vi "Intan_StreamData_64ch_parallelLoop_ambulatory.vi"(0 "VISA resource name":refnum<visa-resource-name>, 1 "refnum in":refnum<file>, 3 "stop streaming":bool, 4 "Save Binary Data":bool, 5 "error in":errorcluster, 7 "byte order":T5(ring)=enum."little-endian", 8 "hdr fpath":path, 11 "DT_scale (sec)":dbl=0.01, 12 "aux file ref num":refnum<file>, 14 "save aux file":bool) -> (6 "N data scans to read (VISA)":i32=20, 10 "Nbytes VISA read":u32, 13 "VISA read iter":i32, 19 "error out":errorcluster)   [LabVIEW 2017]
doc: "Stream data to disk and user friendly display. Data is scaled and filtered prior to display.\n\nThis VI uses parallel while loop architecture: 1 loop reads from serial stream and saves raw bytes to disk; the other loop processes the data in chunk, scaling and filtering, then displays."
uses:
  zip_swcircularbuffer1_0_19b/Circular Buffer/Controls/Circular Buffer Status.ctl
  zip_swcircularbuffer1_0_19b/Circular Buffer/Controls/Circular Buffer Operations.ctl
  <vilib>/Utility/error.llb/DialogType.ctl
  zip_swcircularbuffer1_0_19b/Circular Buffer/Instance VIs/Circular Buffer(1D U16).vi
  zip_swcircularbuffer1_0_19b/Circular Buffer/Circular Buffer.lvlib
panel:
  out "ADXL Stream":dbl[][](graph)
  out "A+B chans":i32[](array[numeric])
  out "Bchans":i32[](array[numeric])
  out "Achans":i32[](array[numeric])
  in  "Tab Control":T1(tab)
  in  "stop logging":bool
  in  "DisplayScale (uV/div)":u16(ring)=1 items=["6400", "3200", "1600", "800", "400", "200", "100", "50", "25"]
  in  "offset factor":dbl=1.0
  in  "Filter settings":T2={"LP Filter On/Off"=TRUE, "LP Cutoff (Hz)"=40.0, "HP Filter On/Off"=TRUE, "HP Cutoff (Hz)"=0.5, "Bandstop On/Off"=TRUE, "fl Cutoff (Hz)"=48.0, "fh Cutoff (Hz) "=52.0}
  out "Save status":bool
  out "non integer read":bool
  out "display iter":i32
  out "% buffer full":dbl(slide) scale=0.0..100.0
  in  "Ring Buffer Size":T3={"Samples per Channel"=640000, "Channels"=0}
  out "buffer underflow":bool
  out "Buffer Status  (read)":T4
  out "buffer overflow":bool
  out "Buffer Status (write)":T4
  in  "Center Traces":bool
  in  "Display Chans":i32[](listbox)=[1, 4, 13, 14, 15, 16, 17, 22]
  out "FS (Hz)":dbl
  in  "ChartDisplayLength (s)":dbl=5.0
  in  "Display Update interval (ms)":dbl=100.0
  in  "Buffer Read Interval (ms)":dbl=100.0
  in  "View Channels":u16(ring) items=["A and B (0-63)", "A chans (0-31)", "B chans (32-63)", "Free Select"]
  in  "bytes per scan":i32=148
  in  "Nchans":i32=64
  in  "start stream (Teensy char)":string="s"
  in  "stop serial stream (Teensy char)":string="t"
  out "Text response":string
  out "timestamp_array":i32[](array[numeric])
  out "aux_cmd_array":i32[][](array[numeric])
  out "binary data (from VISA read)":u16[](array[numeric])
  out "SyncBytes Out":i32[](array[numeric])
  in  "stop logging Teensy char":string="l"
  out "setscaleresult":dbl
  out "UpdateCode":i16
  out "xmax_init":dbl
  out "offset_init":dbl
  out "increment_init":dbl
  out "xmin_init":dbl
  out "NchansChanged":bool
  out "DispLengthChanged":bool
  out "XscaleRollover":bool
  out "error code out":i32 format="%0.0f"
  out "StopLoopsMaster":bool
  out "N_u16s  write to buf":i32
  out "Nelements to read from buf":dbl
  out "N data scans to display":u16=20
  out "YtxtLabelsAll":string[](array[string])
  out "Picture":picture
  out "Intan Streaming Data":dbl[][](graph)
  # "Intan-Teensy Bioelectric Module: Data Stream and Visualization\n64 chan + ADXL"
  # "Data Streaming Frequency"
  # "Display Settings"
  # "Ring Buffer Status"
  # "1-D data stream \nreformatted  to 2-D"
  # "xscale controls"
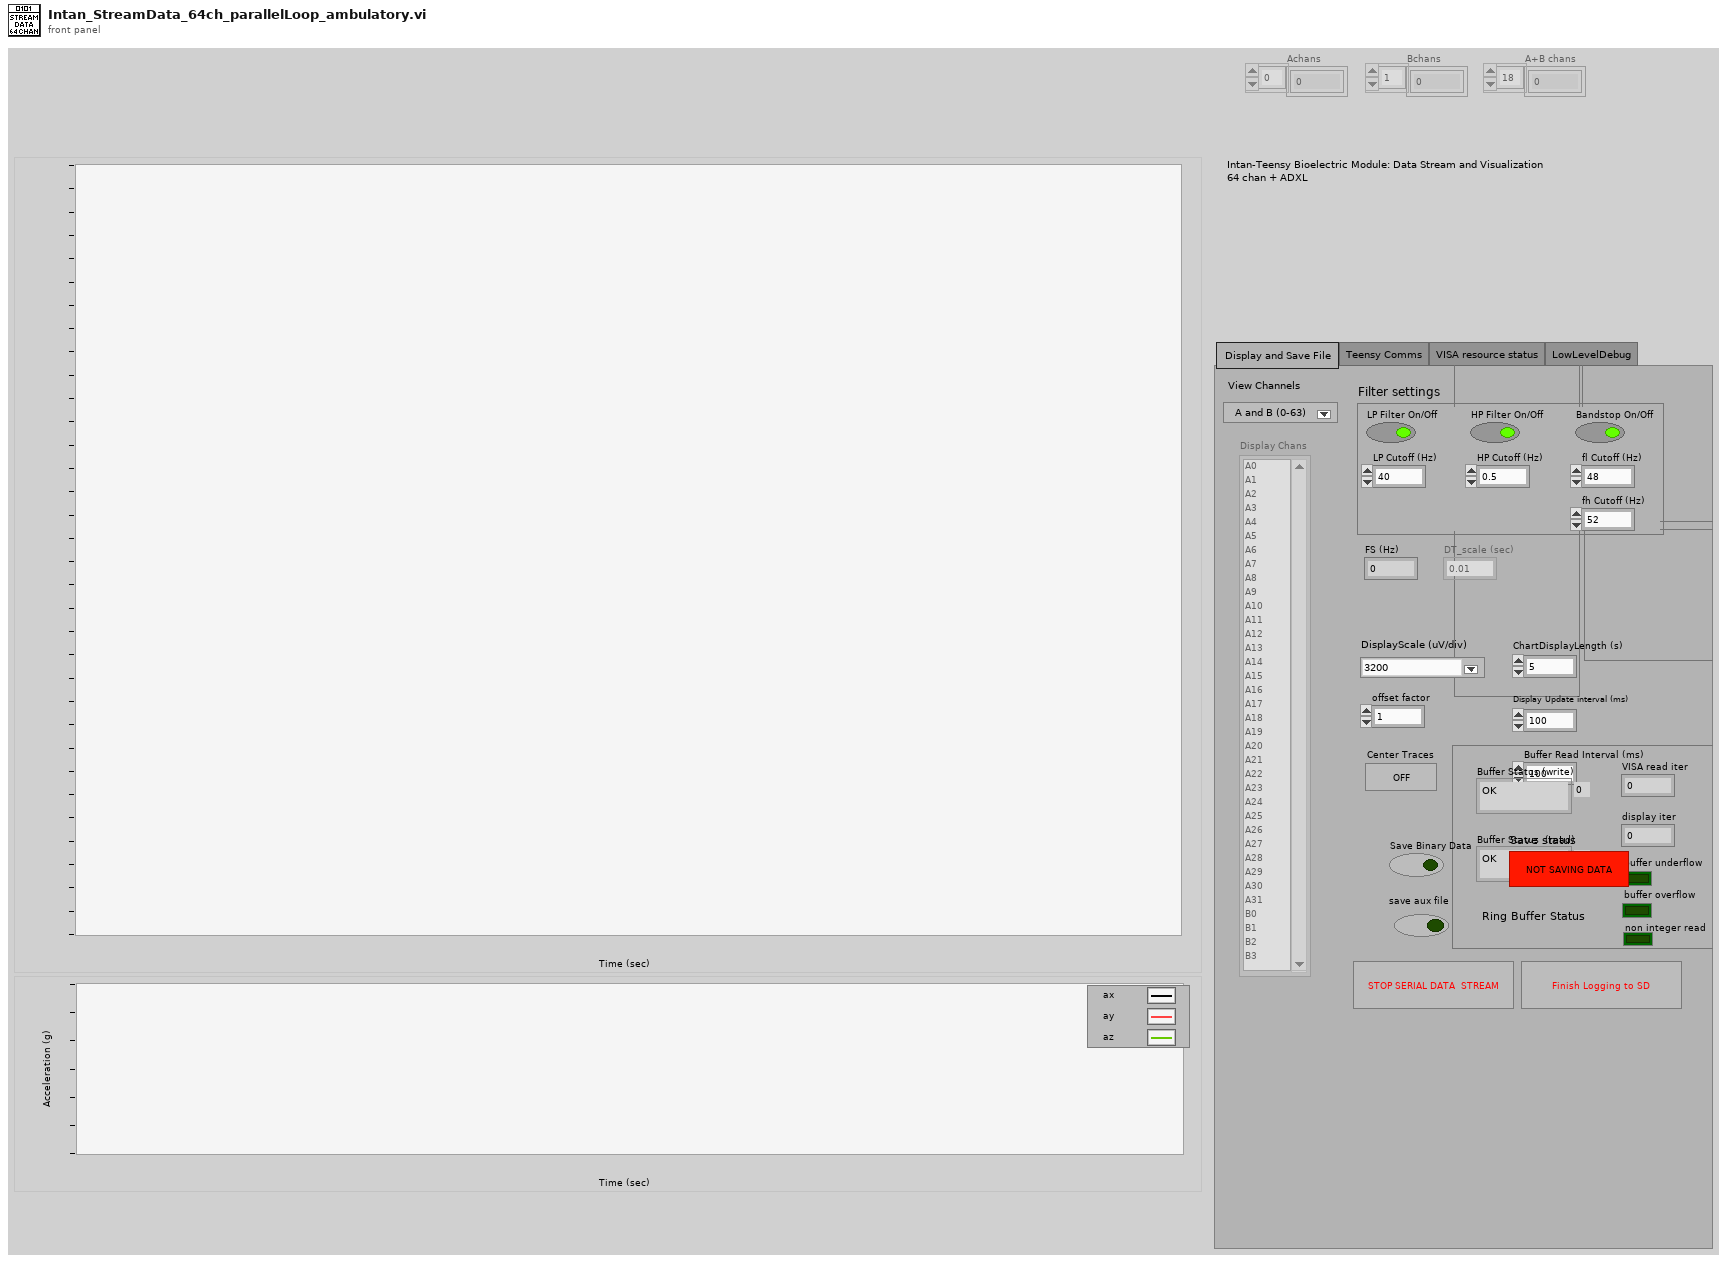
[diagram p1: front panel]
types:
  T1 = enum32{"Display and Save File ", "Teensy Comms", "VISA resource status", "LowLevelDebug"}
  T2 = cluster{"LP Filter On/Off":bool, "LP Cutoff (Hz)":dbl, "HP Filter On/Off":bool, "HP Cutoff (Hz)":dbl, "Bandstop On/Off":bool, "fl Cutoff (Hz)":dbl, "fh Cutoff (Hz) ":dbl}
  T3 = cluster{"Samples per Channel":u32, "Channels":u32}
  T4 = typedef "Circular Buffer.lvlib/Circular Buffer Status.ctl" = enum16{"OK", "Overflow", "Underflow"}
  T5 = enum16{"big-endian, network order", "native, host order", "little-endian"}
  T6 = typedef "Circular Buffer.lvlib/Circular Buffer Operations.ctl" = enum16{"Initialize", "Get Backlog", "Write", "Read (continuous)", "Read (most recent)"}
  T7 = enum8{"Enabled", "Disabled", "Disabled and Grayed Out"}
  T8 = typedef "LVRectTypeDef.ctl" = cluster{"Left":i16, "Top":i16, "Right":i16, "Bottom":i16}
  T9 = cluster{"XScale.Minimum":dbl, "XScale.Maximum":dbl, "XScale.Increment":dbl, "Nchannels":i32}
  T10 = cluster{"Maximum":dbl, dbl, dbl, dbl, dbl, dbl, "YscleMark":dbl, "Increment":dbl}
  T11 = typedef "DialogType.ctl" = u16
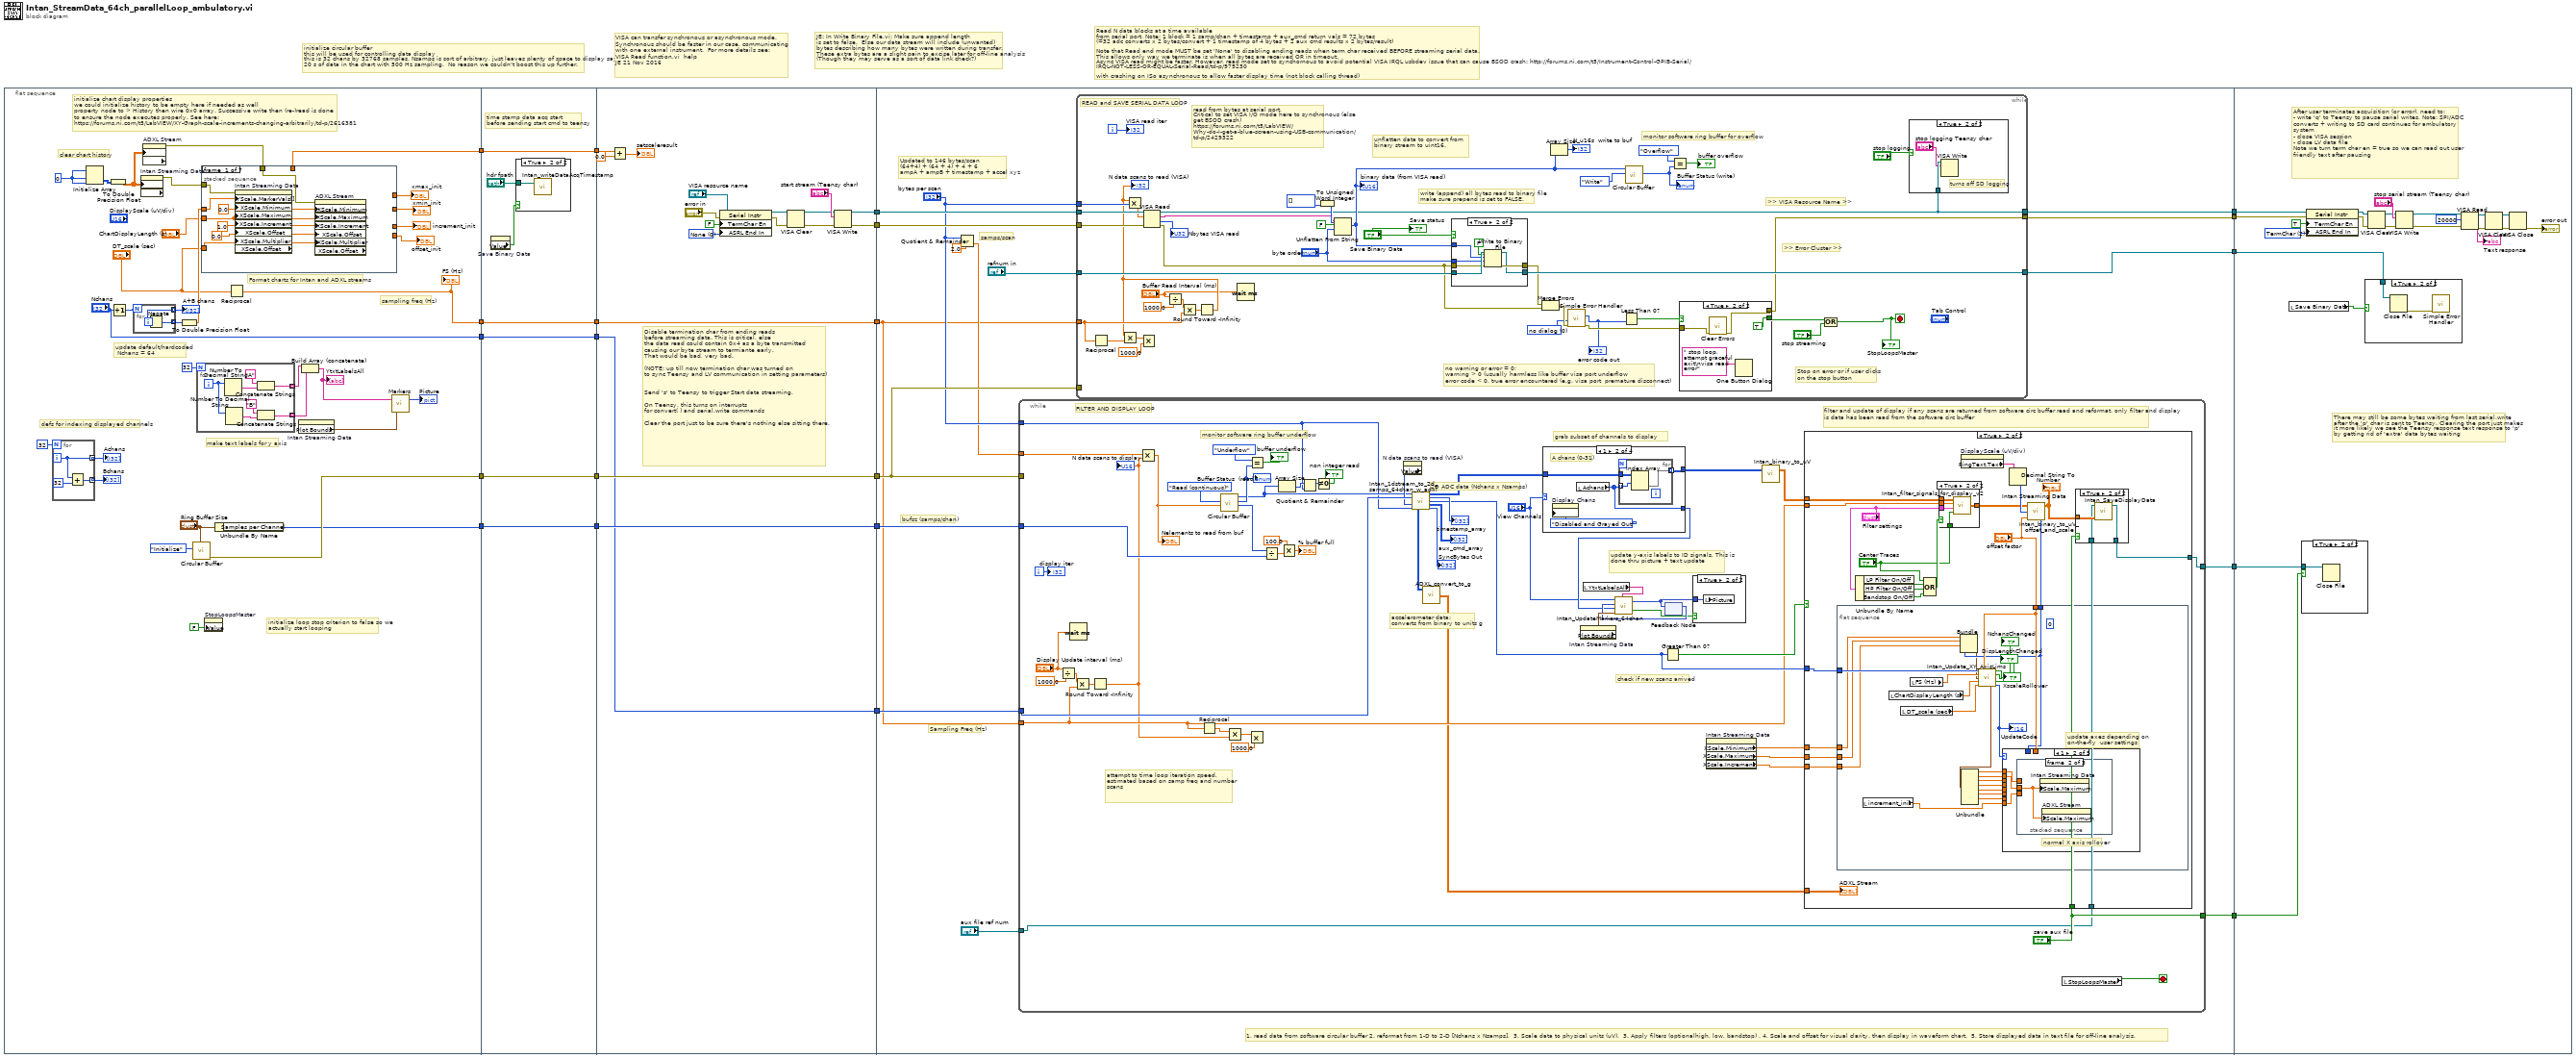
[diagram p0: block diagram]
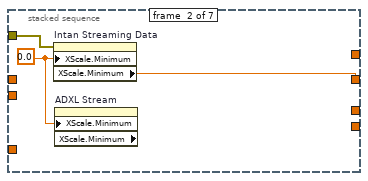
[diagram p2: hidden frame]
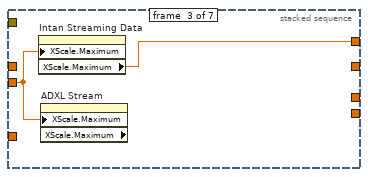
[diagram p3: hidden frame]
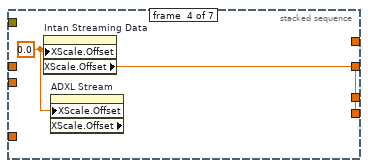
[diagram p4: hidden frame]
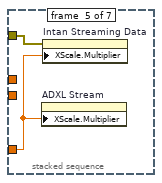
[diagram p5: hidden frame]
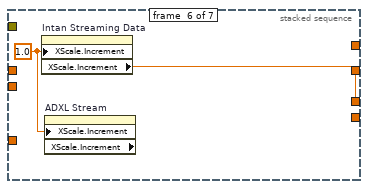
[diagram p6: hidden frame]
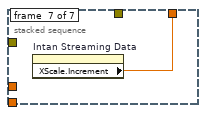
[diagram p7: hidden frame]
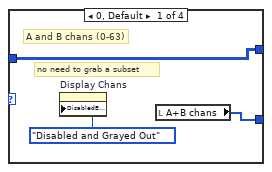
[diagram p10: hidden frame]
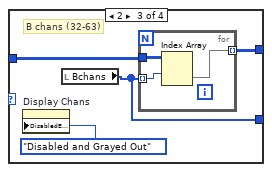
[diagram p11: hidden frame]
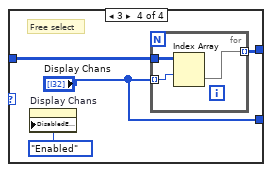
[diagram p12: hidden frame]
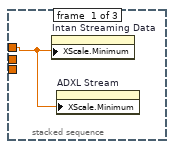
[diagram p15: hidden frame]
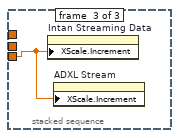
[diagram p16: hidden frame]
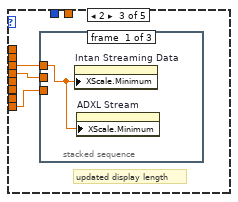
[diagram p17: hidden frame]
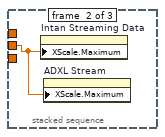
[diagram p18: hidden frame]
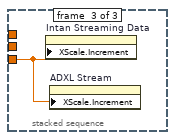
[diagram p19: hidden frame]
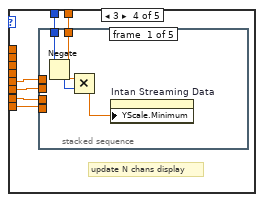
[diagram p20: hidden frame]
diagram:
  # "Read N data blocks at a time available\nfrom serial port. Note: 1 block = 1 samp/chan + timestamp + aux_cmd return vals = 72 bytes \n(=32 adc converts x 2 bytes/convert + 1 timestamp of 4 bytes + 2 aux cmd results x 2 bytes/result) \n\nNote that Read end mode MUST be set 'None' to disabling ending reads when term char received BEFORE streaming serial data.  \nThis allows only way we terminate is when all bytes are received OR in timeout.  \nAsync VISA read might be faster. However, read mode set to synchornous to avoid potential VISA IRQL usbdev issue that can cause BSOD crash: http://forums.ni.com/t5/Instrument-Control-GPIB-Serial/IRQL-NOT-LESS-OR-EQUAL-Serial-Read/td-p/975230\n\nwith crashing on ISo asynchronous to allow faster display time (not block calling thread)"
  # "initialize circular buffer\nthis will be used for controlling data display\nthis is 32 chans by 32768 samples. Nsamps is sort of arbitrary, just leaves plenty of space to display say\n20 s of data in the chart with 500 Hz sampling.  No reason we couldn't boost this up further."
  # "JE: In Write Binary File.vi: Make sure append length \nis set to false.  Else our data stream will include (unwanted)\nbytes describing how many bytes were written during transfer.\nThese extra bytes are a slight pain to excise later for off-line analysis\n(Though they may serve as a sort of data link check?)"
  # "VISA can transfer synchronous or asynchronous mode.\nSynchronous should be faster in our case, communicating\nwith one external instrument.  For more details see: \nVISA Read function.vi  help \nJE 21 Nov 2016"
  n1 = flat-sequence {
    tunnel: [w50] -> w10
    tunnel: [w48] -> w8
    tunnel: ["Nchans"] -> w6
    tunnel: [w43] -> w4
    tunnel: [w32] -> w2
    tunnel: w10 -> [w92]
    tunnel: [w92] -> w9
    tunnel: w8 -> [w91]
    tunnel: [w91] -> w7
    tunnel: w6 -> [w90]
    tunnel: [w90] -> w5
    tunnel: w4 -> [w89]
    tunnel: [w89] -> w3
    tunnel: w2 -> [w88]
    tunnel: [w88] -> w1
    tunnel: [w101] -> w19
    tunnel: [w102] -> w18
    tunnel: [w100] -> w17
    tunnel: w9 -> [w100]
    tunnel: [w99] -> w16
    tunnel: w7 -> [w99]
    tunnel: w5 -> [w98]
    tunnel: [w98] -> w15
    tunnel: [w97] -> w14
    tunnel: w3 -> [w97]
    tunnel: w1 -> [w96]
    tunnel: [w123] -> w21
    tunnel: [w126] -> w20
    tunnel: w19 -> [w124]
    tunnel: w18 -> [w125]
    tunnel: w17 -> [w122]
    tunnel: w16 -> [w120]
    tunnel: w15 -> [w119]
    tunnel: w14 -> [w116]
    tunnel: [w115] -> w13
    tunnel: [w113] -> w12
    tunnel: [w112] -> w11
    tunnel: w21 -> [w370]
    tunnel: w20 -> [w383]
    tunnel: w13 -> [w365]
    tunnel: w12 -> [w364]
    tunnel: w11 -> [w363]
    frame #0 {
      w42 = 0 ("Dimension Size")
      # "Format charts for Intan and ADXL streams"
      # "defs for indexing displayed channels"
      # "update default/hardcoded\n Nchans = 64"
      # "clear chart history"
      # "initialize loop stop criterion to false so we\nactually start looping"
      # "make text labels for y axis"
      # "sampling freq (Hz)"
      # "initialize chart display properties\nwe could initialize history to be empty here if needed as well\nproperty node to > History then wire 0x0 array. Successive write then (re-)read is done\nto ensure the node executes properly. See here:\nhttps://forums.ni.com/t5/LabVIEW/XY-Graph-scale-increments-changing-arbitrarily/td-p/2616381"
      n2 = for {
        N: 32 -> [_]
        tunnel: [w56] -> w30 mode=indexing
        tunnel: [w54] -> w29 mode=indexing
        i -> [w56]
        n3 = Add(x=w56, y=32) -> (x+y=w54:i32)
      }
      "Achans" <- w30
      "Bchans" <- w29
      n4 = Initialize Array(w42, w42, w42) -> (w41:i32[][])
      n5 = To Double Precision Float(number=w41) -> (double precision float=w23:dbl[][])
      n6 = Increment(x="Nchans") -> (x+1=w52:i32)
      n7 = for {
        N: w52 -> [_]
        tunnel: [w85] -> w53 mode=indexing
        tunnel: [w84] -> w28 mode=indexing
        i -> [w84]
        n8 = Negate(x=w84) -> (-x=w85:i32)
      }
      "A+B chans" <- w28
      n9 = property on="Intan Streaming Data" class="WFChart (strict)" props=["History Data", "History Data"]("History Data"=w23) -> (error out=w39:errorcluster)  [unwired: 2 in, 2 out]
      n10 = property on="ADXL Stream" class="WFChart (strict)" props=["History Data", "History Data"]("History Data"=w23) -> (error out=w22:errorcluster)  [unwired: 2 in, 2 out]
      n11 = To Double Precision Float(number=w53) -> (double precision float=w40:dbl[])
      n12 = call-poly "Circular Buffer.vi"("Buffer Size"="Ring Buffer Size", "Operation"=Circular_Buffer_Operations."Initialize") -> ("error out"=w50:errorcluster)  [unwired: 6 in, 3 out]
      n13 = for {
        N: 32 -> [_]
        tunnel: [w81] -> w26 mode=indexing
        tunnel: [w77] -> w25 mode=indexing
        i -> [w78]
        n14 = Number To Decimal String(number=w78) -> (decimal integer string=w83:string)  [unwired: 1 in]
        n15 = Number To Decimal String(number=w78) -> (decimal integer string=w80:string)  [unwired: 1 in]
        n16 = Concatenate Strings("A" ("string"), w83) -> (w81:string)
        n17 = Concatenate Strings("B" ("string"), w80) -> (w77:string)
      }
      n18 = stacked-sequence {
        tunnel: w40 -> [w64 _ _ _ _ _ _]
        tunnel: w39 -> [w63 w66 _ _ w73 _ _]
        tunnel: "ChartDisplayLength (s)" -> [w61 _ w68 _ _ _ _]
        tunnel: "DT_scale (sec)" -> [w58 _ _ _ w72 _ _]
        tunnel: [_ _ w69 _ _ _ _] -> w33
        tunnel: [_ w67 _ _ _ _ _] -> w36
        tunnel: [_ _ _ _ _ w75 _] -> w35
        tunnel: [_ _ _ w71 _ _ _] -> w34
        tunnel: [_ _ _ _ _ _ w76] -> w32
        tunnel: w22 -> [w57 _ _ _ _ _ _]
        frame #0 {
          w60 = 1.0 ("X Scale.Range:Minimum")
          w59 = 0.0 ("X Scale.Range:Minimum")
          w62 = 0.0 ("X Scale.Range:Minimum")
          n19 = property on="Intan Streaming Data" class="WFChart (strict)" props=["YScale", "MarkerVals[]", "XScale", "Minimum", "XScale", "Maximum", "XScale", "Increment", "XScale", "Offset", "XScale", "Multiplier", "XScale", "Offset"](error in=w63, "YScale.MarkerVals[]"=w64, "XScale.Minimum"=w62, "XScale.Maximum"=w61, "XScale.Increment"=w60, "XScale.Offset"=w59, "XScale.Multiplier"=w58) -> ()  [unwired: 1 in, 3 out]
          n20 = property on="ADXL Stream" class="WFChart (strict)" props=["XScale", "Minimum", "XScale", "Maximum", "XScale", "Increment", "XScale", "Offset", "XScale", "Multiplier", "XScale", "Offset"](error in=w57, "XScale.Minimum"=w62, "XScale.Maximum"=w61, "XScale.Increment"=w60, "XScale.Offset"=w59, "XScale.Multiplier"=w58) -> ()  [unwired: 1 in, 3 out]
        }
        frame #1 {
          w65 = 0.0 ("X Scale.Range:Minimum")
          n21 = property on="Intan Streaming Data" class="WFChart (strict)"(error in=w66, "XScale.Minimum"=w65) -> ("XScale.Minimum"=w67:dbl)  [unwired: 1 in, 2 out]
          n22 = property on="ADXL Stream" class="WFChart (strict)" props=["XScale", "Minimum", "XScale", "Minimum"]("XScale.Minimum"=w65) -> ()  [unwired: 2 in, 3 out]
        }
        frame #2 {
          n23 = property on="Intan Streaming Data" class="WFChart (strict)"("XScale.Maximum"=w68) -> ("XScale.Maximum"=w69:dbl)  [unwired: 2 in, 2 out]
          n24 = property on="ADXL Stream" class="WFChart (strict)" props=["XScale", "Maximum", "XScale", "Maximum"]("XScale.Maximum"=w68) -> ()  [unwired: 2 in, 3 out]
        }
        frame #3 {
          w70 = 0.0 ("X Scale.Offset and Multiplier:Offset")
          n25 = property on="Intan Streaming Data" class="WFChart (strict)"("XScale.Offset"=w70) -> ("XScale.Offset"=w71:dbl)  [unwired: 2 in, 2 out]
          n26 = property on="ADXL Stream" class="WFChart (strict)" props=["XScale", "Offset", "XScale", "Offset"]("XScale.Offset"=w70) -> ()  [unwired: 2 in, 3 out]
        }
        frame #4 {
          n27 = property on="ADXL Stream" class="WFChart (strict)"("XScale.Multiplier"=w72) -> ()  [unwired: 2 in, 2 out]
          n28 = property on="Intan Streaming Data" class="WFChart (strict)"(error in=w73, "XScale.Multiplier"=w72) -> ()  [unwired: 1 in, 2 out]
        }
        frame #5 {
          w74 = 1.0 ("X Scale.Range:Increment")
          n29 = property on="Intan Streaming Data" class="WFChart (strict)"("XScale.Increment"=w74) -> ("XScale.Increment"=w75:dbl)  [unwired: 2 in, 2 out]
          n30 = property on="ADXL Stream" class="WFChart (strict)" props=["XScale", "Increment", "XScale", "Increment"]("XScale.Increment"=w74) -> ()  [unwired: 2 in, 3 out]
        }
        frame #6 {
          n31 = property on="Intan Streaming Data" class="WFChart (strict)"() -> ("XScale.Increment"=w76:dbl)  [unwired: 2 in, 2 out]
        }
      }
      "xmin_init" <- w36
      "increment_init" <- w35
      "offset_init" <- w34
      "xmax_init" <- w33
      n32 = property on="StopLoopsMaster" class="Bool (strict)"("Value"=FALSE ("StopLoopsMaster")) -> ()  [unwired: 2 in, 2 out]
      n33 = Unbundle By Name("Ring Buffer Size") -> ("Samples per Channel"=w48:u32)
      n34 = Reciprocal(x="DT_scale (sec)") -> (1/x=w43:dbl)
      "FS (Hz)" <- w43
      n35 = property on="Intan Streaming Data" class="WFChart (strict)"() -> ("Plot Bounds"=w44:T8)  [unwired: 2 in, 2 out]
      n36 = Build Array (concatenate)(w26, w25) -> (w24:string[])
      "YtxtLabelsAll" <- w24
      n37 = call "Markers.vi"("plot bounds"=w44, "Array"=w24) -> ("Picture"=→"Picture":picture)  [unwired: 1 out]
    }
    frame #1 {
      # "time stamp data acq start\nbefore sending start cmd to teensy"
      n38 = property on="Save Binary Data" class="Bool (strict)"() -> ("Value"=w87:bool)  [unwired: 2 in, 2 out]
      n39 = case shown="True" w87 {
        tunnel: "hdr fpath" -> [_ w93]
        frame False {
        }
        frame True {
          n40 = call "Intan_writeDataAcqTimestamp.vi"("hdr fpath"=w93) -> ()  [unwired: 2 in, 1 out]
        }
      }
    }
    frame #2 {
      w107 = u16 0 items=["None", "Last Bit", "TermChar"] ("Serial Settings:End Mode for Reads")
      # "Disable termination char from ending reads\nbefore streaming data. This is critical, else\nthe data read could contain 0x4 as a byte transmitted\ncausing our byte stream to termiante early.\nThat would be bad, very bad.\n\n(NOTE: up till now termination char was turned on\nto sync Teensy and LV communication in setting parameters)\n\n\nSend 's' to Teensy to trigger Start data streaming.  \n\nOn Teensy, this turns on interrupts\nfor convert( ) and serial.write commands\n\nClear the port just to be sure there's nothing else sitting there."
      n41 = Add(x=w96, y=0.0) -> (x+y=→"setscaleresult":dbl)
      n42 = property class="Serial Instr"(reference="VISA resource name", error in="error in", "TermChar En"=FALSE ("Message Based Settings:Termination Character Enable"), "ASRL End In"=w107) -> (reference out=w106:refnum<visa-resource-name>, error out=w105:errorcluster)
      n43 = VISA Clear(VISA resource name=w106, error in (no error)=w105) -> (VISA resource name out=w104:refnum<visa-resource-name>, error out=w103:errorcluster)
      n44 = VISA Write(VISA resource name=w104, write buffer="start stream (Teensy char)", error in (no error)=w103) -> (VISA resource name out=w102:refnum<visa-resource-name>, error out=w101:errorcluster)  [unwired: 1 out]
    }
    frame #3 {
      # "Updated to 146 bytes/scan\n(64+4) + (64 + 4) + 4 + 6\nampA + ampB + timestamp + accel xyz"
      # "1. read data from software circular buffer 2. reformat from 1-D to 2-D [Nchans x Nsamps].  3. Scale data to physical units (uV).  3. Apply filters (optionalhigh, low, bandstop) . 4. Scale and offset for visual clarity, then display in waveform chart.  5. Store displayed data in text file for off-line analysis."
      # "Sampling Freq (Hz)"
      # "bufsz (samps/chan)"
      # "samps/scan"
      n45 = Quotient & Remainder(x="bytes per scan", y=2.0) -> (floor(x/y)=w117:dbl)  [unwired: 1 out]
      n46 = while {
        tunnel: w122 -> [_]
        tunnel: w120 -> [w174]
        tunnel: w119 -> [w170]
        tunnel: "bytes per scan" -> [w160]
        tunnel: w116 -> [w141]
        tunnel: w117 -> [w166]
        tunnel: [w147] -> w115
        tunnel: "aux file ref num" -> [w146]
        tunnel: ["save aux file"] -> w112
        i -> [w167]
        stop <- w144 stop-if-true
        # "accelerometer data: \nconverts from binary to units g"
        # "2D ADC data (Nchans x Nsamps)"
        # "check if new scans arrived"
        # "grab subset of channels to display"
        # "update y-axis labels to ID signals. This is done thru picture + text update"
        # "FILTER AND DISPLAY LOOP"
        # "attempt to time loop iteration speed,\nestimated based on samp freq and number scans"
        # "filter and update of display if any scans are returned from software circ buffer read and reformat. only filter and display is data has been read from the software circ buffer"
        # "monitor software ring buffer underflow"
        n47 = Divide(x="Display Update interval (ms)", y=1000.0) -> (x/y=w138:dbl)
        n48 = Wait (ms)(milliseconds to wait="Display Update interval (ms)") -> ()  [unwired: 1 out]
        n49 = Multiply(x=w138, y=w141) -> (x*y=w140:dbl)
        n50 = Round Toward -Infinity(1:w140) -> (0:w139:dbl)
        "N data scans to display" <- w139
        n51 = Multiply(x=w166, y=w139) -> (x*y=w165:dbl)
        "Nelements to read from buf" <- w165
        n52 = Reciprocal(x=w141) -> (1/x=w157:dbl)
        n53 = call-poly "Circular Buffer.vi"("Read Size"=w165, "Operation"=Circular_Buffer_Operations."Read (continuous)") -> ("Elements Remaining"=w175:i32, "Buffer Status"=w177:T4, "Data Out"=w162:u16[])  [unwired: 6 in, 1 out]
        "Buffer Status  (read)" <- w177
        n54 = Multiply(x=w157, y=w139) -> (x*y=w156:dbl)
        n55 = Multiply(x=w156, y=1000.0) -> ()  [unwired: 1 out]
        n56 = Equal?(x=Circular_Buffer_Status."Underflow" ("y"), y=w177) -> (x = y?=→"buffer underflow":bool)
        n57 = Divide(x=w175, y=w174) -> (x/y=w173:dbl)
        n58 = Array Size(array=w162) -> (size(s)=w161:i32)
        n59 = Multiply(x=100.0, y=w173) -> (x*y=→"% buffer full":dbl)
        n60 = Quotient & Remainder(x=w161, y=w160) -> (x-y*floor(x/y)=w159:i32)  [unwired: 1 out]
        n61 = Not Equal To 0?(x=w159) -> (x != 0?=→"non integer read":bool)
        n62 = property on="N data scans to read (VISA)" class="DigNum (strict)"() -> ("Value"=w164:i32)  [unwired: 2 in, 2 out]
        n63 = call "Intan_1dstream_to_2d_samps_64chan_w_adxl.vi"("1-D  data in"=w162, "Nchans"=w170, "N data scans to read"=w164, "bytes per scan"=w160) -> ("2d ADCdata_array out_ampA_and_B"=w154:u16[][], "timestamp_array"=→"timestamp_array":i32[], "Nscans read"=w145:i32, "aux_cmd_array A_and_B"=→"aux_cmd_array":i16[][], "ADXL analog data out"=w130:u16[][], "SyncBytes Out"=→"SyncBytes Out":i32[])  [unwired: 4 in, 2 out]
        n64 = call "ADXL_convert_to_g.vi"("ADXL analog data out: Binary format"=w130) -> ("ADXL scaled (units of g)"=w129:dbl[][])  [unwired: 3 in]
        n65 = case shown="1" "View Channels" {
          tunnel: w154 -> [w183 w187 w194 w201]
          tunnel: [w183 w186 w193 w200] -> w143
          tunnel: [w181 w184 w191 "Display Chans"] -> w132
          frame 0, Default {
            # "A and B chans (0-63)"
            # "no need to grab a subset"
            n66 = property on="Display Chans" class="LstBox (strict)"("DisabledEnum"=T7."Disabled and Grayed Out" ("Disabled")) -> ()  [unwired: 2 in, 2 out]
            n67 = local read "A+B chans"() -> (w181:i32[])
          }
          frame 1 {
            # "A chans (0-31)"
            n68 = property on="Display Chans" class="LstBox (strict)"("DisabledEnum"=T7."Disabled and Grayed Out" ("Disabled")) -> ()  [unwired: 2 in, 2 out]
            n69 = local read "Achans"() -> (w184:i32[])
            n70 = for {
              tunnel: w187 -> [w190]
              tunnel: w184 -> [w188] mode=indexing
              tunnel: [w189] -> w186 mode=indexing
              n71 = Index Array(array=w190, index (row)=w188) -> (element=w189:u16[])  [unwired: 1 in]
            }
          }
          frame 2 {
            # "B chans (32-63)"
            n72 = property on="Display Chans" class="LstBox (strict)"("DisabledEnum"=T7."Disabled and Grayed Out" ("Disabled")) -> ()  [unwired: 2 in, 2 out]
            n73 = local read "Bchans"() -> (w191:i32[])
            n74 = for {
              tunnel: w194 -> [w197]
              tunnel: w191 -> [w195] mode=indexing
              tunnel: [w196] -> w193 mode=indexing
              n75 = Index Array(array=w197, index (row)=w195) -> (element=w196:u16[])  [unwired: 1 in]
            }
          }
          frame 3 {
            # "Free select"
            n76 = property on="Display Chans" class="LstBox (strict)"("DisabledEnum"=T7."Enabled" ("Disabled")) -> ()  [unwired: 2 in, 2 out]
            n77 = for {
              tunnel: w201 -> [w204]
              tunnel: "Display Chans" -> [w202] mode=indexing
              tunnel: [w203] -> w200 mode=indexing
              n78 = Index Array(array=w204, index (row)=w202) -> (element=w203:u16[])  [unwired: 1 in]
            }
          }
        }
        n79 = property on="Intan Streaming Data" class="WFChart (strict)"() -> ("Plot Bounds"=w152:T8)  [unwired: 2 in, 2 out]
        n80 = local read "YtxtLabelsAll"() -> (w142:string[])
        n81 = Greater Than 0?(x=w145) -> (x > 0?=w163:bool)
        n82 = feedback #1() -> (w151:picture)  [unwired: 1 in]
        n83 = call "Intan_UpdateMarkers_64chan.vi"("ChanSelectMode"="View Channels", "Picture In"=w151, "Display Chans"=w132, "plot bounds"=w152, "YtxtLabelsAll"=w142) -> ("Picture Out"=w149:picture, "update labels"=w150:bool)
        n84 = feedback-in #1(w149) -> ()
        n85 = case shown="True" w150 {
          tunnel: w149 -> [_ w180]
          frame False {
          }
          frame True {
            n86 = local write "Picture"(w180) -> ()
          }
        }
        n87 = property on="Intan Streaming Data" class="WFChart (strict)"() -> ("XScale.Minimum"=w135:dbl, "XScale.Maximum"=w134:dbl, "XScale.Increment"=w133:dbl)  [unwired: 2 in, 2 out]
        n88 = call "Intan_binary_to_uV.vi"("2d ADC binary data"=w143) -> ("Scaled Data (uV)"=w153:dbl[][])  [unwired: 2 in]
        n89 = case shown="True" w163 {
          tunnel: w141 -> [_ w226]
          tunnel: w153 -> [_ w224]
          tunnel: [w205 w217] -> w147
          tunnel: "save aux file" -> [_ w216]
          tunnel: w146 -> [w205 w215]
          tunnel: w145 -> [_ w213]
          tunnel: w135 -> [_ w209]
          tunnel: w134 -> [_ w208]
          tunnel: w133 -> [_ w207]
          tunnel: w129 -> [_ w206]
          frame False {
          }
          frame True {
            n90 = flat-sequence {
              tunnel: w213 -> [w248]
              tunnel: "offset factor" -> [w235]
              tunnel: w210 -> [w232]
              tunnel: w209 -> [w230]
              tunnel: w208 -> [w229]
              tunnel: w207 -> [w228]
              frame #0 {
                (unwired) 0 ("index")
                # "update axes depending on\non-the-fly  user settings"
                n91 = local read "increment_init"() -> (w234:dbl)
                n92 = local read "ChartDisplayLength (s)"() -> (w246:dbl)
                n93 = local read "DT_scale (sec)"() -> (w245:dbl)
                n94 = local read "FS (Hz)"() -> (w247:dbl)
                n95 = Bundle("XScale.Minimum"=w230, "XScale.Maximum"=w229, "XScale.Increment"=w228, "Nchannels"=w232) -> (w231:T9)  [unwired: 1 in]
                n96 = call "Intan_Update_XY_AxisLims.vi"("NscansRead"=w248, "offset factor"=w235, "FS (Hz)"=w247, "XscaleClusterCurrent"=w231, "DisplayLength(s)"=w246, "DT_scale (s)"=w245) -> ("XscaleRollover"=→"XscaleRollover":bool, "DispLengthChanged"=→"DispLengthChanged":bool, "NchansChanged"=→"NchansChanged":bool, "XYlims Update Cluster"=w243:T10, "UpdateCode"=w244:i16)  [unwired: 4 in, 1 out]
                "UpdateCode" <- w244
                n97 = Unbundle(w243) -> ("Maximum"=w240:dbl, w239:dbl, w237:dbl, w236:dbl, w242:dbl, w241:dbl, "YscleMark"=w238:dbl)  [unwired: 1 out]
                n98 = case shown="1" w244 {
                  tunnel: w232 -> [_ _ _ w268 w279]
                  tunnel: w242 -> [_ _ _ w263 _]
                  tunnel: w241 -> [_ _ _ w267 _]
                  tunnel: w240 -> [_ w253 _ _ w282]
                  tunnel: w239 -> [_ w252 _ _ w281]
                  tunnel: w238 -> [_ _ _ w266 w280]
                  tunnel: w237 -> [_ _ w258 _ _]
                  tunnel: w236 -> [_ _ w259 _ _]
                  tunnel: w235 -> [_ _ _ w265 w278]
                  tunnel: w234 -> [_ w251 w257 w264 w277]
                  frame 0, Default {
                    # "nothing to update"
                  }
                  frame 1 {
                    # "normal X axis rollover"
                    n99 = stacked-sequence {
                      tunnel: w253 -> [w254 _ _]
                      tunnel: w252 -> [_ w255 _]
                      tunnel: w251 -> [_ _ w256]
                      frame #0 {
                        n100 = property on="Intan Streaming Data" class="WFChart (strict)"("XScale.Minimum"=w254) -> ()  [unwired: 2 in, 2 out]
                        n101 = property on="ADXL Stream" class="WFChart (strict)"("XScale.Minimum"=w254) -> ()  [unwired: 2 in, 2 out]
                      }
                      frame #1 {
                        n102 = property on="Intan Streaming Data" class="WFChart (strict)"("XScale.Maximum"=w255) -> ()  [unwired: 2 in, 2 out]
                        n103 = property on="ADXL Stream" class="WFChart (strict)"("XScale.Maximum"=w255) -> ()  [unwired: 2 in, 2 out]
                      }
                      frame #2 {
                        n104 = property on="Intan Streaming Data" class="WFChart (strict)"("XScale.Increment"=w256) -> ()  [unwired: 2 in, 2 out]
                        n105 = property on="ADXL Stream" class="WFChart (strict)"("XScale.Increment"=w256) -> ()  [unwired: 2 in, 2 out]
                      }
                    }
                  }
                  frame 2 {
                    # "updated display length"
                    n106 = stacked-sequence {
                      tunnel: w257 -> [_ _ w262]
                      tunnel: w259 -> [_ w261 _]
                      tunnel: w258 -> [w260 _ _]
                      frame #0 {
                        n107 = property on="Intan Streaming Data" class="WFChart (strict)"("XScale.Minimum"=w260) -> ()  [unwired: 2 in, 2 out]
                        n108 = property on="ADXL Stream" class="WFChart (strict)"("XScale.Minimum"=w260) -> ()  [unwired: 2 in, 2 out]
                      }
                      frame #1 {
                        n109 = property on="Intan Streaming Data" class="WFChart (strict)"("XScale.Maximum"=w261) -> ()  [unwired: 2 in, 2 out]
                        n110 = property on="ADXL Stream" class="WFChart (strict)"("XScale.Maximum"=w261) -> ()  [unwired: 2 in, 2 out]
                      }
                      frame #2 {
                        n111 = property on="Intan Streaming Data" class="WFChart (strict)"("XScale.Increment"=w262) -> ()  [unwired: 2 in, 2 out]
                        n112 = property on="ADXL Stream" class="WFChart (strict)"("XScale.Increment"=w262) -> ()  [unwired: 2 in, 2 out]
                      }
                    }
                  }
                  frame 3 {
                    # "update N chans display"
                    n113 = stacked-sequence {
                      tunnel: w268 -> [w272 _ _ _ _]
                      tunnel: w264 -> [_ _ _ _ w276]
                      tunnel: w267 -> [_ _ _ w275 _]
                      tunnel: w266 -> [_ _ _ _ _]
                      tunnel: w265 -> [w270 _ _ _ _]
                      tunnel: w263 -> [_ w273 w274 _ _]
                      frame #0 {
                        n114 = Negate(x=w272) -> (-x=w271:i32)
                        n115 = Multiply(x=w270, y=w271) -> (x*y=w269:dbl)
                        n116 = property on="Intan Streaming Data" class="WFChart (strict)"("YScale.Minimum"=w269) -> ()  [unwired: 2 in, 2 out]
                      }
                      frame #1 {
                        n117 = property on="Intan Streaming Data" class="WFChart (strict)"("XScale.Offset"=w273) -> ()  [unwired: 2 in, 2 out]
                      }
                      frame #2 {
                        n118 = property on="Intan Streaming Data" class="WFChart (strict)"("XScale.Minimum"=w274) -> ()  [unwired: 2 in, 2 out]
                      }
                      frame #3 {
                        n119 = property on="Intan Streaming Data" class="WFChart (strict)"("XScale.Maximum"=w275) -> ()  [unwired: 2 in, 2 out]
                      }
                      frame #4 {
                        n120 = property on="Intan Streaming Data" class="WFChart (strict)"("XScale.Increment"=w276) -> ()  [unwired: 2 in, 2 out]
                      }
                    }
                  }
                  frame 4 {
                    # "updated offset factor"
                    n121 = stacked-sequence {
                      seq-local: [w283 _ _] -> [_ w287 _]
                      tunnel: w282 -> [_ _ _]
                      tunnel: w281 -> [_ _ _]
                      tunnel: w280 -> [_ _ _]
                      tunnel: w279 -> [w286 _ _]
                      tunnel: w278 -> [w284 _ _]
                      tunnel: w277 -> [_ _ w292]
                      frame #0 {
                        n122 = Negate(x=w286) -> (-x=w285:i32)
                        n123 = Multiply(x=w284, y=w285) -> (x*y=w283:dbl)
                        n124 = property on="Intan Streaming Data" class="WFChart (strict)"("YScale.Minimum"=w283) -> ()  [unwired: 2 in, 2 out]
                      }
                      frame #1 {
                        n125 = for {
                          N: w287 -> [_]
                          tunnel: [w290] -> w289 mode=indexing
                          i -> [w291]
                          n126 = Negate(x=w291) -> (-x=w290:i32)
                        }
                        n127 = To Double Precision Float(number=w289) -> (double precision float=w288:dbl[])
                        n128 = property on="Intan Streaming Data" class="WFChart (strict)" props=["YScale", "MarkerVals[]", "YScale", "MarkerVals[]"]("YScale.MarkerVals[]"=w288) -> ()  [unwired: 2 in, 3 out]
                      }
                      frame #2 {
                        n129 = property on="Intan Streaming Data" class="WFChart (strict)"("XScale.Increment"=w292) -> ()  [unwired: 2 in, 2 out]
                      }
                    }
                  }
                }
              }
            }
            n130 = Unbundle By Name("Filter settings") -> ("LP Filter On/Off"=w222:bool, "HP Filter On/Off"=w221:bool, "Bandstop On/Off"=w219:bool)
            n131 = Compound Arithmetic op=OR("Center Traces", w222, w221, w219) -> (w220:bool)
            n132 = case shown="True" w220 {
              tunnel: w226 -> [_ w302]
              tunnel: w224 -> [w297 w301]
              tunnel: [w297 w300] -> w214
              tunnel: "Filter settings" -> [_ w299]
              tunnel: "Center Traces" -> [_ w298]
              frame False {
              }
              frame True {
                n133 = call "Intan_filter_signals_for_display_v2.vi"("Center Traces"=w298, "input filter cluster"=w299, "Sample Rate (Hz)"=w302, "Nchan Array In [Nchans x Nsamps]"=w301) -> ("Display Signals Out [Nchans x Nsamps]"=w300:dbl[][])
              }
            }
            n134 = property on="DisplayScale (uV/div)" class="Ring (strict)"() -> ("RingText.Text"=w225:string)  [unwired: 2 in, 2 out]
            n135 = Decimal String To Number(string=w225) -> (number=w227:i32)  [unwired: 2 in, 1 out]
            n136 = call "Intan_binary_to_uV_offset_and_scale.vi"("offset spacing factor"="offset factor", "Yscale (uv/div)"=w227, "ScaledData [Nchans x Nsamps]"=w214) -> ("Nchannels"=w210:i32, "Data4Display"=w212:dbl[][])  [unwired: 1 in]
            "Intan Streaming Data" <- w212
            n137 = case shown="True" w216 {
              tunnel: w212 -> [_ w296]
              tunnel: [w293 w295] -> w217
              tunnel: w215 -> [w293 w294]
              frame False {
              }
              frame True {
                n138 = call "Intan_SaveDisplayData.vi"("2d ADCdata_array out"=w296, "aux file ref num"=w294) -> ("refnum out"=w295:refnum<file>)  [unwired: 3 in]
              }
            }
            "ADXL Stream" <- w206
          }
        }
        n139 = local read "StopLoopsMaster"() -> (w144:bool)
        "display iter" <- w167
      }
      n140 = while {
        tunnel: [w304] -> w123
        tunnel: [w343] -> w126
        tunnel: w124 -> [w339]
        tunnel: "refnum in" -> [w342]
        tunnel: w125 -> [w340]
        tunnel: w122 -> [_]
        tunnel: "bytes per scan" -> [w324]
        tunnel: w116 -> [w307]
        tunnel: [w311] -> w113
        i -> [w341]
        stop <- w344 stop-if-true
        w317 = T11 0 items=["no dialog", "OK message", "continue or stop message", "OK message + warnings", "continue/stop + warnings"] ("type of dialog (OK msg:1)")
        # "no warning or error = 0;\nwarning > 0 (usually harmless like buffer visa port underflow\nerror code < 0, true error encountered (e.g. visa port  premature disconnect)"
        # "READ and SAVE SERIAL DATA LOOP"
        # "monitor software ring buffer for overflow"
        # "write (append) all bytes read to binary file\nmake sure prepend is set to FALSE."
        # "unflatten data to convert from binary stream to uint16."
        # "Stop on error or if user clicks \non the stop button"
        # ">> Error Cluster >>"
        # ">> VISA Resource Name >>"
        # "read from bytes at serial port.\nCritical to set VISA I/O mode here to synchronous (else get BSOD crash)\nhttps://forums.ni.com/t5/LabVIEW/Why-do-I-get-a-blue-screen-using-USB-communication/td-p/2429322"
        n141 = Reciprocal(x=w307) -> (1/x=w321:dbl)
        n142 = Divide(x="Buffer Read Interval (ms)", y=1000.0) -> (x/y=w309:dbl)
        n143 = Multiply(x=w309, y=w307) -> (x*y=w310:dbl)
        n144 = Round Toward -Infinity(1:w310) -> (0:w306:dbl)
        "N data scans to read (VISA)" <- w306
        n145 = Multiply(x=w306, y=w321) -> (x*y=w323:dbl)
        n146 = Multiply(x=w306, y=w324) -> (x*y=w325:dbl)
        n147 = Multiply(x=w323, y=1000.0) -> ()  [unwired: 1 out]
        n148 = VISA Read(VISA resource name=w340, byte count=w325, error in (no error)=w339) -> (VISA resource name out=w304:refnum<visa-resource-name>, read buffer=w333:string, return count=→"Nbytes VISA read":u32, error out=w319:errorcluster)
        n149 = Wait (ms)(milliseconds to wait="Buffer Read Interval (ms)") -> ()  [unwired: 1 out]
        n150 = To Unsigned Word Integer(number=i16[] []) -> (unsigned 16bit integer=w335:u16[])
        n151 = Unflatten From String(type=w335, binary string=w333, data includes array or string size? (T)=FALSE, byte order (0:big-endian, network order)="byte order") -> (value=w327:u16[])  [unwired: 1 in, 2 out]
        "binary data (from VISA read)" <- w327
        n152 = case shown="True" "Save Binary Data" {
          tunnel: [w354 w361] -> w320
          tunnel: [w353 w360] -> w343
          tunnel: w342 -> [w353 w359]
          tunnel: w319 -> [w354 w358]
          tunnel: "byte order" -> [_ w356]
          tunnel: w327 -> [_ w355]
          frame False {
          }
          frame True {
            n153 = Write to Binary File(file (use dialog)=w359, data=w355, error in=w358, 5:FALSE ("prepend array or string size? (T)"), 9:w356) -> (refnum out=w360:refnum<file>, error out=w361:errorcluster)  [unwired: 1 in, 1 out]
          }
        }
        n154 = Merge Errors(w320, w319) -> (w318:errorcluster)
        n155 = Array Size(array=w327) -> (size(s)=→"N_u16s  write to buf":i32)
        n156 = call <vilib>:"Simple Error Handler.vi"("type of dialog (OK msg:1)"=w317, "error in (no error)"=w318) -> ("code out"=w314:i32, "error out"=w315:errorcluster)  [unwired: 3 in, 3 out]
        "error code out" <- w314
        n157 = Less Than 0?(x=w314) -> (x < 0?=w312:bool)
        n158 = call-poly "Circular Buffer.vi"("Operation"=Circular_Buffer_Operations."Write", "Data In"=w327) -> ("Buffer Status"=w329:T4)  [unwired: 6 in, 3 out]
        "Buffer Status (write)" <- w329
        n159 = Equal?(x=Circular_Buffer_Status."Overflow" ("y"), y=w329) -> (x = y?=→"buffer overflow":bool)
        n160 = case shown="True" w312 {
          tunnel: w315 -> [w347 w351]
          tunnel: [FALSE TRUE] -> w313
          tunnel: [w347 w349] -> w311
          frame False {
          }
          frame True {
            n161 = call <vilib>:"Clear Errors.vi"("error in (no error)"=w351) -> ("error out"=w349:errorcluster)  [unwired: 5 in, 1 out]
            n162 = One Button Dialog(message=" stop loop, attempt graceful exit\nvisa read error") -> ()  [unwired: 1 in, 1 out]
          }
        }
        n163 = Compound Arithmetic op=OR(w313, "stop streaming") -> (w344:bool)
        "StopLoopsMaster" <- w344
        n164 = case shown="True" "stop logging" {
          tunnel: w304 -> [_ w346]
          frame False {
          }
          frame True {
            # "turns off SD logging"
            n165 = VISA Write(VISA resource name=w346, write buffer="stop logging Teensy char") -> ()  [unwired: 1 in, 3 out]
          }
        }
        "VISA read iter" <- w341
        "Save status" <- "Save Binary Data"
      }
    }
    frame #4 {
      w375 = u16 2 items=["None", "Last Bit", "TermChar"] ("Serial Settings:End Mode for Reads")
      # "There may still be some bytes waiting from last serial.write\nafter the 'p' char is sent to Teensy. Clearing the port just makes\nit more likely we see the Teensy response text response to 'p' \nby getting rid of 'extra' data bytes waiting"
      # "After user terminates acquisition (or error), need to:\n- write 'q' to Teensy to pause serial writes. Note: SPI/ADC converts + writing to SD card continues for ambulatory system\n- close VISA session\n- close LV data file\nNote we turn term char en = true so we can read out user friendly text after pausing"
      n166 = local read "Save Binary Data"() -> (w362:bool)
      n167 = case shown="True" w363 {
        tunnel: w365 -> [_ w386]
        frame False {
        }
        frame True {
          n168 = Close File(refnum=w386) -> ()  [unwired: 1 in, 2 out]
        }
      }
      n169 = property class="Serial Instr"(reference=w370, error in=w364, "TermChar En"=TRUE ("Message Based Settings:Termination Character Enable"), "ASRL End In"=w375) -> (reference out=w369:refnum<visa-resource-name>, error out=w368:errorcluster)
      n170 = case shown="True" w362 {
        tunnel: w383 -> [_ w384]
        frame False {
        }
        frame True {
          n171 = Close File(refnum=w384) -> (error out=w385:errorcluster)  [unwired: 1 in, 1 out]
          n172 = call <vilib>:"Simple Error Handler.vi"("error in (no error)"=w385) -> ()  [unwired: 4 in, 5 out]
        }
      }
      n173 = VISA Clear(VISA resource name=w369, error in (no error)=w368) -> (VISA resource name out=w367:refnum<visa-resource-name>, error out=w366:errorcluster)
      n174 = VISA Write(VISA resource name=w367, write buffer="stop serial stream (Teensy char)", error in (no error)=w366) -> (VISA resource name out=w378:refnum<visa-resource-name>, error out=w377:errorcluster)  [unwired: 1 out]
      n175 = VISA Read(VISA resource name=w378, byte count=u32 20000, error in (no error)=w377) -> (VISA resource name out=w374:refnum<visa-resource-name>, read buffer=→"Text response":string, error out=w372:errorcluster)  [unwired: 1 out]
      n176 = VISA Clear(VISA resource name=w374, error in (no error)=w372) -> (VISA resource name out=w373:refnum<visa-resource-name>, error out=w371:errorcluster)
      n177 = VISA Close(VISA resource name=w373, error in (no error)=w371) -> (error out=→"error out":errorcluster)
    }
  }
